vi "主程序.vi"() -> ()   [LabVIEW 2012]
panel:
  out "暂无传送门":bool
  out "得分":i32
  out "地图名称":enum16{"无迷宫", "方盒", "铁道", "工厂"}(ring)
  out "点":cluster{"x":dbl, "y":dbl}={"x"=1.0, "y"=10.0}
  out "地图":u32[][](array[colorbox])
  out "方向":enum16{"左", "右", "上", "下"}(ring)
  out "蛇":cluster{"x":dbl, "y":dbl}[](array[cluster])
  out "状态":bool=TRUE
  out "行列数":i32
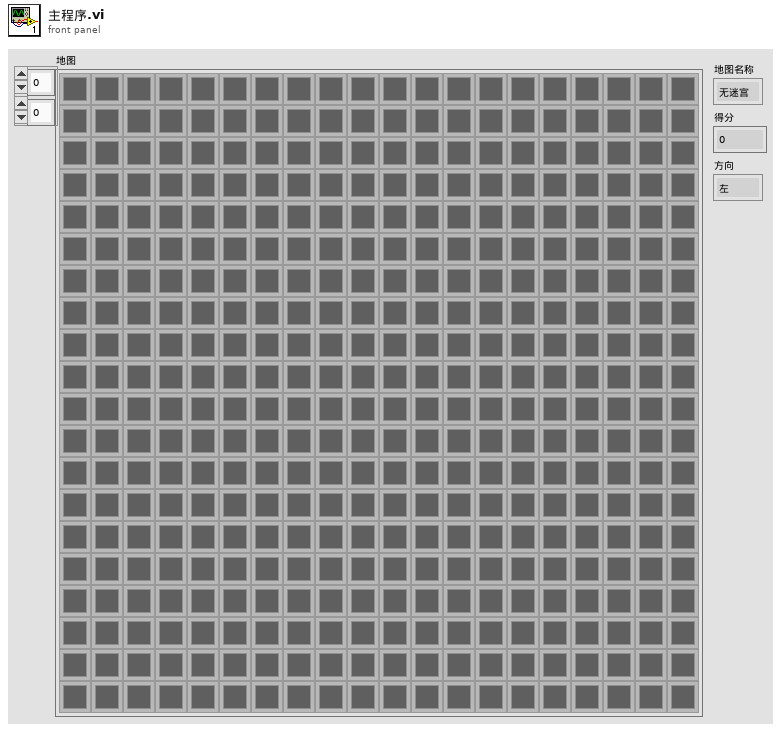
[diagram p1: front panel]
types:
  T1 = typedef "eventvkey.ctl" = enum16{"ASCII", "Enter", "Return", "Shift", "Ctrl", "Alt", "Cmd", "Opt", "Caps", "NumLock", "Clear", "Break", "Up", "Down", "Left", "Right", "Insert", "Delete", "Home", "End", "PageUp", "PageDown", "Escape", "Help", "Pause", "ScrollLock", "F1", "F2", "F3", "F4", "F5", "F6", "F7", "F8", "F9", "F10", "F11", "F12", "F13", "F14", "F15", "F16", "F17", "F18", "F19", "F20", "F21", "F22", "F23", "F24", "Play", "VolumeUp", "VolumeDown", "Mute", "Two Byte Char"}
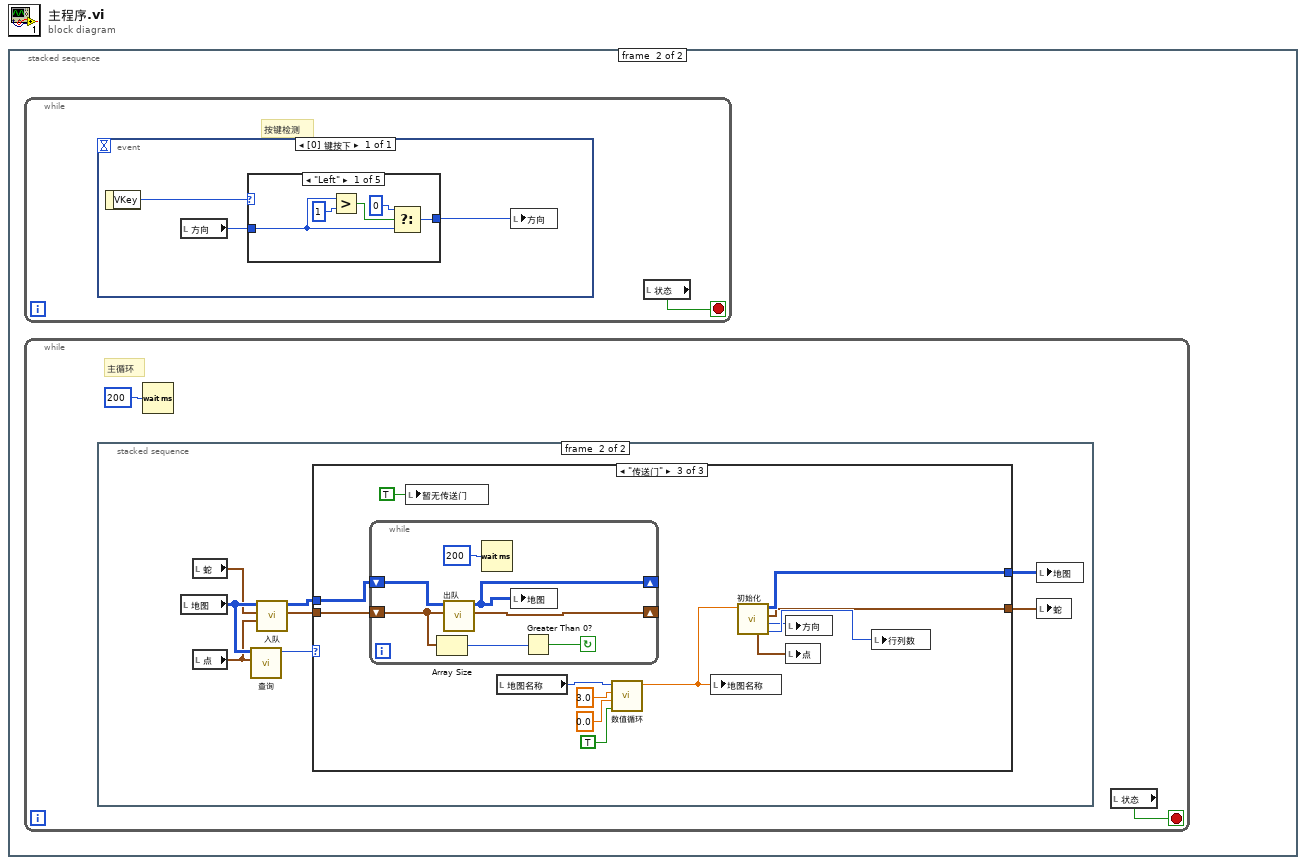
[diagram p0: block diagram]
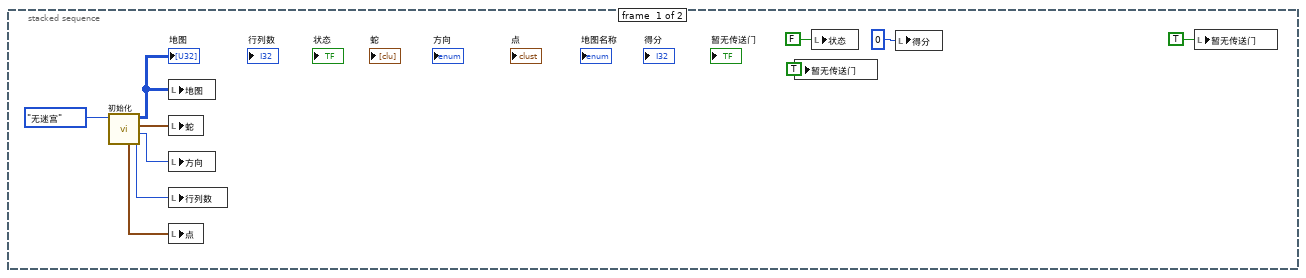
[diagram p2: hidden frame]
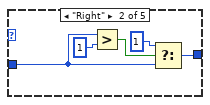
[diagram p3: hidden frame]
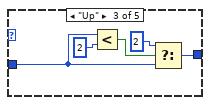
[diagram p4: hidden frame]
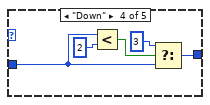
[diagram p5: hidden frame]
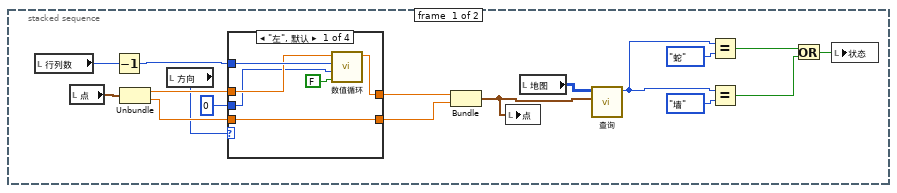
[diagram p7: hidden frame]
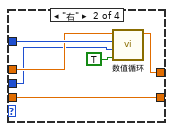
[diagram p8: hidden frame]
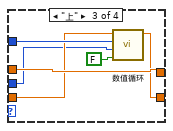
[diagram p9: hidden frame]
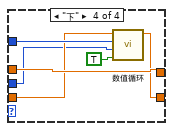
[diagram p10: hidden frame]
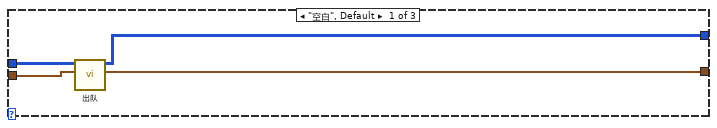
[diagram p11: hidden frame]
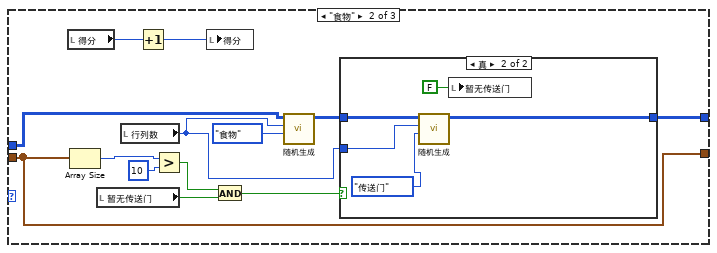
[diagram p12: hidden frame]
diagram:
  n1 = stacked-sequence {
    frame #0 {
      n2 = call "初始化.vi"("地图编号"=enum16{"无迷宫", "方盒", "铁道", "工厂"}."无迷宫") -> ("行列数"=w8:i32, "方向"=w6:enum16{"左", "右", "上", "下"}, "蛇"=w7:cluster{"x":dbl, "y":dbl}[], "地图"=w5:u32[][], "初始位置"=w4:cluster{"x":dbl, "y":dbl})  [unwired: 6 in]
      "地图" <- w5
      n3 = local write "地图"(w5) -> ()
      n4 = local write "蛇"(w7) -> ()
      n5 = local write "方向"(w6) -> ()
      n6 = local write "行列数"(w8) -> ()
      n7 = local write "点"(w4) -> ()
      n8 = local write "暂无传送门"(TRUE ("状态")) -> ()
      n9 = local write "状态"(FALSE ("状态")) -> ()
      n10 = local write "得分"(0) -> ()
      n11 = local write "暂无传送门"(TRUE ("状态")) -> ()
    }
    frame #1 {
      n12 = while {
        stop <- w11 stop-if-true
        # "按键检测"
        n13 = event shown="[0] 键按下" {
          selector: _ -> [_]
          dyn-events: _ -> [_]
          timeout: _ -> [_]
          event Key Down {
            n14 = event-data() -> ("VKey"=w14:T1)  [unwired: 1 in]
            n15 = local read "方向"() -> (w13:enum16{"左", "右", "上", "下"})
            n16 = case shown="\"Left\"" w14 {
              tunnel: w13 -> [w16 w21 w26 w31 w35]
              tunnel: [w15 w20 w25 w30 w35] -> w12
              frame "Left" {
                n17 = Greater?(x=w16, y=1) -> (0:w18:bool)
                n18 = Select(t=u16 0, s=w18, f=w16) -> (s? t:f=w15:u16)
              }
              frame "Right" {
                n19 = Greater?(x=w21, y=1) -> (0:w23:bool)
                n20 = Select(t=u16 1, s=w23, f=w21) -> (s? t:f=w20:u16)
              }
              frame "Up" {
                n21 = Less?(x=w26, y=2) -> (x < y?=w28:bool)
                n22 = Select(t=u16 2, s=w28, f=w26) -> (s? t:f=w25:u16)
              }
              frame "Down" {
                n23 = Less?(x=w31, y=2) -> (x < y?=w33:bool)
                n24 = Select(t=u16 3, s=w33, f=w31) -> (s? t:f=w30:u16)
              }
              frame "ASCII", Default {
              }
            }
            n25 = local write "方向"(w12) -> ()
          }
        }
        n26 = local read "状态"() -> (w11:bool)
      }
      n27 = while {
        stop <- w36 stop-if-true
        # "主循环"
        n28 = stacked-sequence {
          frame #0 {
            n29 = local read "行列数"() -> (w51:i32)
            n30 = local read "点"() -> (w54:cluster{"x":dbl, "y":dbl})
            n31 = Decrement(x=w51) -> (x-1=w38:i32)
            n32 = Unbundle(w54) -> ("x"=w53:dbl, "y"=w52:dbl)
            n33 = local read "方向"() -> (w50:enum16{"左", "右", "上", "下"})
            n34 = case shown="\"左\", 默认" w50 {
              tunnel: w53 -> [w57 w62 w70 w76]
              tunnel: w52 -> [w58 w65 w69 w75]
              tunnel: [w56 w63 w70 w76] -> w49
              tunnel: [w58 w65 w68 w74] -> w48
              tunnel: w38 -> [w59 w64 w71 w77]
              tunnel: 0 -> [w55 w61 w67 w73]
              frame "左", Default {
                n35 = call "数值循环.vi"("加/减"=FALSE, "下限"=w55, "上限"=w59, "输入"=w57) -> ("输出"=w56:dbl)  [unwired: 7 in]
              }
              frame "右" {
                n36 = call "数值循环.vi"("加/减"=TRUE, "下限"=w61, "上限"=w64, "输入"=w62) -> ("输出"=w63:dbl)  [unwired: 7 in]
              }
              frame "上" {
                n37 = call "数值循环.vi"("加/减"=FALSE, "下限"=w67, "上限"=w71, "输入"=w69) -> ("输出"=w68:dbl)  [unwired: 7 in]
              }
              frame "下" {
                n38 = call "数值循环.vi"("加/减"=TRUE, "下限"=w73, "上限"=w77, "输入"=w75) -> ("输出"=w74:dbl)  [unwired: 7 in]
              }
            }
            n39 = Bundle("x"=w49, "输出"=w48) -> (w46:cluster{"x":dbl, "输出":dbl})  [unwired: 1 in]
            n40 = local write "点"(w46) -> ()
            n41 = local read "地图"() -> (w47:u32[][])
            n42 = call "查询.vi"("点"=w46, "地图"=w47) -> ("索引1"=w45:enum16{"空白", "蛇", "食物", "墙", "传送门"})  [unwired: 9 in]
            n43 = Equal?(x=w45, y=enum16{"空白", "蛇", "食物", "墙", "传送门"}."蛇" ("索引1")) -> (x = y?=w41:bool)
            n44 = Equal?(x=w45, y=enum16{"空白", "蛇", "食物", "墙", "传送门"}."墙" ("值")) -> (x = y?=w42:bool)
            n45 = Or(x=w41, y=w42) -> (x .or. y?=w40:bool)
            n46 = local write "状态"(w40) -> ()
          }
          frame #1 {
            n47 = local read "地图"() -> (w86:u32[][])
            n48 = local read "蛇"() -> (w85:cluster{"x":dbl, "y":dbl}[])
            n49 = local read "点"() -> (w84:cluster{"x":dbl, "y":dbl})
            n50 = call "查询.vi"("点"=w84, "地图"=w86) -> ("索引1"=w83:enum16{"空白", "蛇", "食物", "墙", "传送门"})  [unwired: 9 in]
            n51 = call "入队.vi"("输入点"=w84, "数组输入"=w85, "地图"=w86) -> ("数组输出"=w81:cluster{"x":dbl, "y":dbl}[], "地图 2"=w82:u32[][])  [unwired: 7 in]
            n52 = case shown="\"传送门\"" w83 {
              tunnel: w82 -> [w90 w103 w122]
              tunnel: w81 -> [w89 w101 w121]
              tunnel: [w88 w92 w113] -> w80
              tunnel: [w87 w101 w112] -> w79
              frame "空白", Default {
                n53 = call "出队.vi"("数组输入"=w89, "地图"=w90) -> ("数组输出"=w87:cluster{"x":dbl, "y":dbl}[], "地图 2"=w88:u32[][])  [unwired: 8 in]
              }
              frame "食物" {
                n54 = local read "得分"() -> (w98:i32)
                n55 = Array Size(array=w101) -> (size(s)=w100:i32)
                n56 = local read "暂无传送门"() -> (w91:bool)
                n57 = local read "行列数"() -> (w94:i32)
                n58 = Increment(x=w98) -> (x+1=w97:i32)
                n59 = Greater?(x=w100, y=10) -> (0:w96:bool)
                n60 = local write "得分"(w97) -> ()
                n61 = And(x=w96, y=w91) -> (x .and. y?=w95:bool)
                n62 = call "随机生成.vi"("类型"=enum16{"空白", "蛇", "食物", "墙", "传送门"}."食物", "上限"=w94, "地图"=w103) -> ("地图 2"=w93:u32[][])  [unwired: 8 in]
                n63 = case shown="真" w95 {
                  tunnel: w94 -> [_ w109]
                  tunnel: w93 -> [w104 w108]
                  tunnel: [w104 w107] -> w92
                  frame False {
                  }
                  frame True {
                    n64 = call "随机生成.vi"("类型"=enum16{"空白", "蛇", "食物", "墙", "传送门"}."传送门", "上限"=w109, "地图"=w108) -> ("地图 2"=w107:u32[][])  [unwired: 8 in]
                    n65 = local write "暂无传送门"(FALSE ("暂无传送门")) -> ()
                  }
                }
              }
              frame "传送门" {
                n66 = while {
                  shift-right: [w126] -> _
                  shift-left: w121 -> [w127]
                  shift-right: [w124] -> _
                  shift-left: w122 -> [w125]
                  stop <- w128 continue-if-true
                  n67 = Array Size(array=w127) -> (size(s)=w129:i32)
                  n68 = call "出队.vi"("数组输入"=w127, "地图"=w125) -> ("数组输出"=w126:cluster{"x":dbl, "y":dbl}[], "地图 2"=w124:u32[][])  [unwired: 8 in]
                  n69 = Wait (ms)(milliseconds to wait=u32 200 ("等待时间（毫秒）")) -> ()  [unwired: 1 out]
                  n70 = local write "地图"(w124) -> ()
                  n71 = Greater Than 0?(x=w129) -> (x > 0?=w128:bool)
                }
                n72 = local write "暂无传送门"(TRUE ("已有传送门")) -> ()
                n73 = local read "地图名称"() -> (w120:enum16{"无迷宫", "方盒", "铁道", "工厂"})
                n74 = call "数值循环.vi"("加/减"=TRUE, "下限"=0.0, "上限"=3.0, "输入"=w120) -> ("输出"=w111:dbl)  [unwired: 7 in]
                n75 = local write "地图名称"(w111) -> ()
                n76 = call "初始化.vi"("地图编号"=w111) -> ("行列数"=w115:i32, "方向"=w114:enum16{"左", "右", "上", "下"}, "蛇"=w112:cluster{"x":dbl, "y":dbl}[], "地图"=w113:u32[][], "初始位置"=w116:cluster{"x":dbl, "y":dbl})  [unwired: 6 in]
                n77 = local write "方向"(w114) -> ()
                n78 = local write "点"(w116) -> ()
                n79 = local write "行列数"(w115) -> ()
              }
            }
            n80 = local write "地图"(w80) -> ()
            n81 = local write "蛇"(w79) -> ()
          }
        }
        n82 = Wait (ms)(milliseconds to wait=u32 200 ("等待时间（毫秒）")) -> ()  [unwired: 1 out]
        n83 = local read "状态"() -> (w36:bool)
      }
    }
  }
